vi "Init.vi"(8 "error in":errorcluster, 11 "Tool Tip Text in":refnum<class "Tool Tip Text.lvclass">) -> (0 "error out":errorcluster, 3 "Tool Tip Text out":refnum<class "Tool Tip Text.lvclass">)   [LabVIEW 2023, in "SourceGrid.lvlib" / "Tool Tip Text.lvclass"]
uses:
  Tool Tip Text.lvclass
  Tool Tip Text.lvclass/Tool Tip Text.ctl
  D:/git/Sourcegrid-LabVIEW/dll/SourceGrid.dll
  dll/SourceGrid.dll
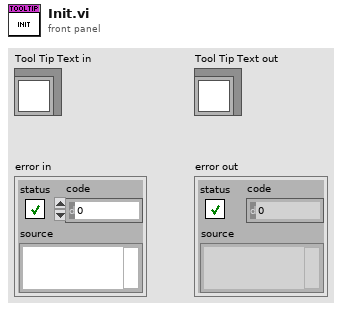
[diagram p1: front panel]
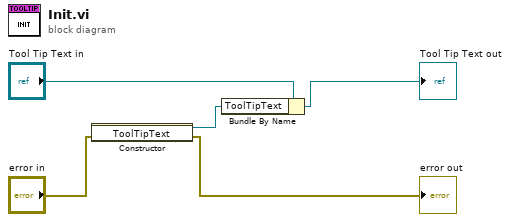
[diagram p0: block diagram]
diagram:
  n1 = constructor class="ToolTipText"(error in="error in") -> (reference out=w2:refnum<k24>, error out=→"error out":errorcluster)  [unwired: 2 in, 1 out]
  n2 = Bundle By Name(cluster="Tool Tip Text in", "ToolTipText"=w2) -> (→"Tool Tip Text out":refnum<class "Tool Tip Text.lvclass">)
